vi "AlarmCalculateLevelsResponse_Parse.vi"(8 "error in (no error)":errorcluster, 11 "Message":T7) -> (0 "error out":errorcluster, 1 "Body":T1, 2 "Header":T6, 3 "AlarmCalculateLevelsResponse":T5)   [LabVIEW 2017]
uses:
  <vilib>/addons/InsightCM/MessageBus/Base/controls/Message.ctl
  <vilib>/addons/InsightCM/MessageBus/Base/controls/MessageHeader.ctl
  <vilib>/addons/InsightCM/MessageBus/Base/controls/KeyValuePair.ctl
  <vilib>/addons/InsightCM/MessageBus/MessageLibrary/TrendAlarm/controls/AlarmCalculateLevelsResponse.ctl
  <vilib>/addons/InsightCM/MessageBus/MessageLibrary/TrendAlarm/controls/AlarmCalculateLevelsResponseBody.ctl
  <vilib>/addons/InsightCM/MessageBus/Base/controls/TrendAlarmLevel.ctl
  <vilib>/addons/InsightCM/MessageBus/Base/controls/AlarmAction.ctl
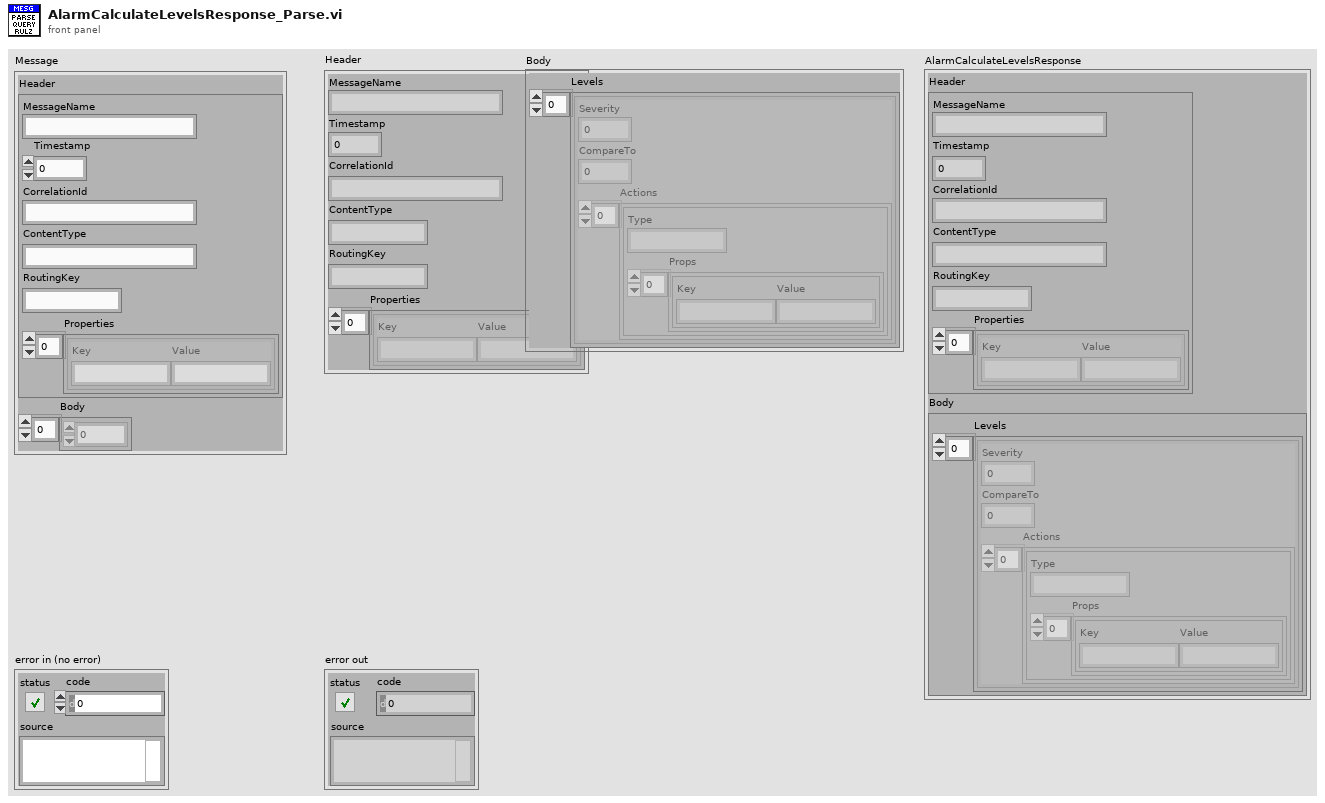
[diagram p1: front panel]
types:
  T1 = typedef "AlarmCalculateLevelsResponseBody.ctl" = cluster{"Levels":T2[]}
  T2 = typedef "TrendAlarmLevel.ctl" = cluster{"Severity":i32, "CompareTo":dbl, "Actions":T3[]}
  T3 = typedef "AlarmAction.ctl" = cluster{"Type":string, "Props":T4[]}
  T4 = typedef "KeyValuePair.ctl" = cluster{"Key":string, "Value":string}
  T5 = typedef "AlarmCalculateLevelsResponse.ctl" = cluster{"Header":T6, "Body":T1}
  T6 = typedef "MessageHeader.ctl" = cluster{"MessageName":string, "Timestamp":i64, "CorrelationId":string, "ContentType":string, "RoutingKey":string, "Properties":T4[]}
  T7 = typedef "Message.ctl" = cluster{"Header":T6, "Body":u8[]}
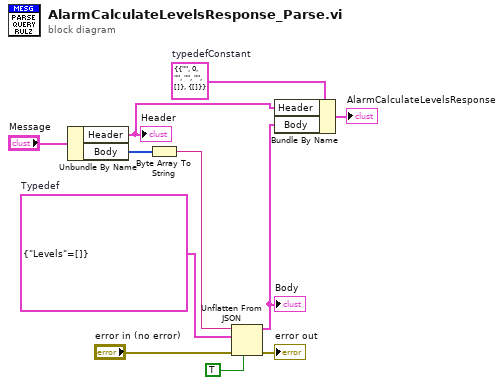
[diagram p0: block diagram]
diagram:
  w3 = T5 {"Header"={"MessageName"="", "Timestamp"=0, "CorrelationId"="", "ContentType"="", "RoutingKey"="", "Properties"=[]}, "Body"={"Levels"=[]}}  # typedefConstant
  w7 = T1 {"Levels"=[]}  # Typedef
  n1 = Unbundle By Name("Message") -> ("Header"=w9:T6, "Body"=w1:u8[])
  "Header" <- w9
  n2 = Byte Array To String(unsigned byte array=w1) -> (string=w6:string)
  n3 = Unflatten From JSON(JSON string=w6, type and defaults=w7, default null elements? (F)=TRUE, error in (no error)="error in (no error)") -> (value=w5:T1, error out=→"error out":errorcluster)  [unwired: 3 in]
  "Body" <- w5
  n4 = Bundle By Name(cluster=w3, "Header"=w9, "Body"=w5) -> (→"AlarmCalculateLevelsResponse":T5)
